vi "epx_Update.vi"(6 "Background Decoratin":refnum<vi>, 7 "Vector Diagram":refnum<vi>, 8 "error in (no error)":errorcluster, 9 "Container State":T3, 10 "Display State In":T1={"BGColor"=0, "FGColor"=0, "GridColor"=9868950, "Number of Polar Grids"=12, "Number of Circle Grids"=4, "Vector.Active"=0, "Vectors.Properties"=[], "Height"=0, "Width"=0} {"Number of Circle Grids" min=1 max=100 step=1; "Number of Polar Grids" min=1 max=100 step=1}, 11 "Data In":T4) -> (0 "error out":errorcluster, 2 "Display State Out":T1={"BGColor"=0, "FGColor"=0, "GridColor"=9868950, "Number of Polar Grids"=12, "Number of Circle Grids"=4, "Vector.Active"=0, "Vectors.Properties"=[], "Height"=0, "Width"=0} {"Number of Circle Grids" min=1 max=100 step=1; "Number of Polar Grids" min=1 max=100 step=1})   [LabVIEW 2011, in "NI_EP_Basic.lvlib" / "EPX Vector Diagram.xctl"]
uses:
  <vilib>/addons/Electrical Power/Basic/Controls/Vector Diagram/EPX Vector Diagram.xctl
  <vilib>/addons/Electrical Power/Basic/Controls/Vector Diagram/Abilities/epx_Vector Diagram State.ctl
  <vilib>/addons/Electrical Power/Basic/Controls/Vector Diagram/SubVIs/epx_Vector Type.ctl
  <vilib>/addons/Electrical Power/Basic/Controls/Vector Diagram/Abilities/epx_Vector Diagram Data.ctl
  <vilib>/_xctls/Container State.ctl
  <vilib>/addons/Electrical Power/Basic/NI_EP_Basic.lvlib
  <vilib>/_xctls/XControlSupport.lvlib
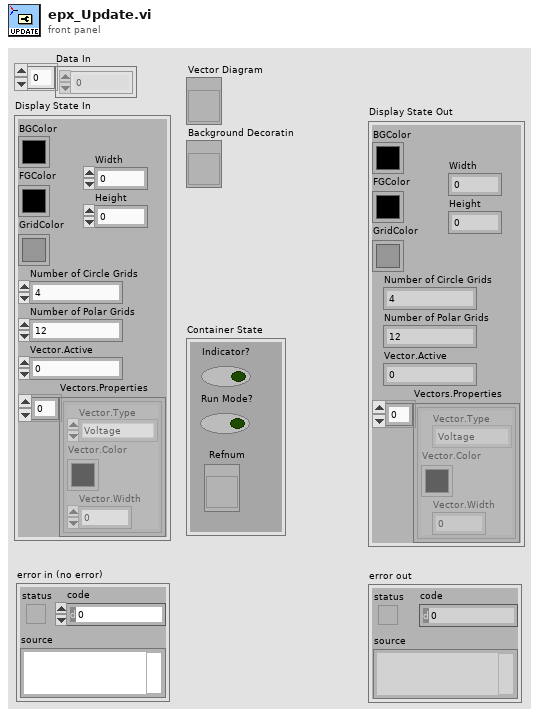
[diagram p1: front panel]
types:
  T1 = typedef "NI_EP_Basic.lvlib/EPX Vector Diagram.xctl/epx_Vector Diagram State.ctl" = cluster{"BGColor":u32, "FGColor":u32, "GridColor":u32, "Number of Polar Grids":i32, "Number of Circle Grids":i32, "Vector.Active":i32, "Vectors.Properties":cluster{"Vector.Type":T2, "Vector.Color":u32, "Vector.Width":u8}[], "Height":u32, "Width":u32}
  T2 = typedef "NI_EP_Basic.lvlib/epx_Vector Type.ctl" = enum16{"Voltage", "Current"}
  T3 = typedef "XControlSupport.lvlib/Container State.ctl" = cluster{"Indicator?":bool, "Run Mode?":bool, " Refnum":refnum<vi>}
  T4 = typedef "NI_EP_Basic.lvlib/EPX Vector Diagram.xctl/epx_Vector Diagram Data.ctl" = cdb[]
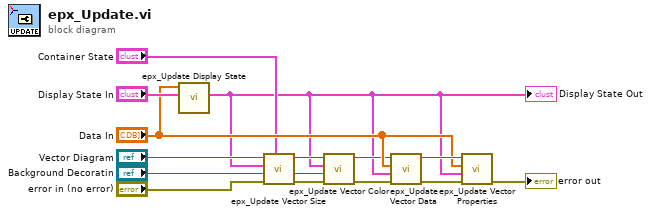
[diagram p0: block diagram]
diagram:
  n1 = call <vilib>:"epx_Update Display State.vi"("Display State In"="Display State In", "Data In"="Data In") -> ("Display State Out"=w1:T1)  [unwired: 8 in, 1 out]
  "Display State Out" <- w1
  n2 = call <vilib>:"epx_Update Vector Size.vi"("Container State"="Container State", "error in (no error)"="error in (no error)", "Background Decoratin"="Background Decoratin", "Display State In"=w1, "Vector Diagram"="Vector Diagram") -> ("error out"=w4:errorcluster, "Background Decoratin out"=w2:refnum<vi>, "Vector Diagram out"=w6:refnum<vi>)  [unwired: 4 in]
  n3 = call <vilib>:"epx_Update Vector Color.vi"("error in (no error)"=w4, "Background Decoratin"=w2, "Display State In"=w1, "Vector Diagram"=w6) -> ("error out"=w3:errorcluster, "Vector Diagram out"=w5:refnum<vi>)  [unwired: 5 in, 1 out]
  n4 = call <vilib>:"epx_Update Vector Data.vi"("error in (no error)"=w3, "Display State In"=w1, "Data In"="Data In", "Vector Diagram"=w5) -> ("error out"=w13:errorcluster, "Vector Diagram out"=w14:refnum<vi>)  [unwired: 6 in]
  n5 = call <vilib>:"epx_Update Vector Properties.vi"("error in (no error)"=w13, "Display State In"=w1, "Data In"="Data In", "Vector Diagram"=w14) -> ("error out"=→"error out":errorcluster)  [unwired: 6 in, 1 out]
